vi "Test Status Correct on Added Method.vi"(8 "error in (no error)":errorcluster, 11 "Result Model Tests in":refnum<class "Result Model Test Enumeration.lvclass">) -> (0 "error out":errorcluster, 3 "Result Model Tests out":refnum<class "Result Model Test Enumeration.lvclass">)   [LabVIEW 2020, in "Result Model Test Enumeration.lvclass"]
uses:
  Result Model Test Enumeration.lvclass
  source/User Interface/Result Model/Result Model.lvclass
  206db1ee-aa99-40b9-8881-171f2a77c34b.vi
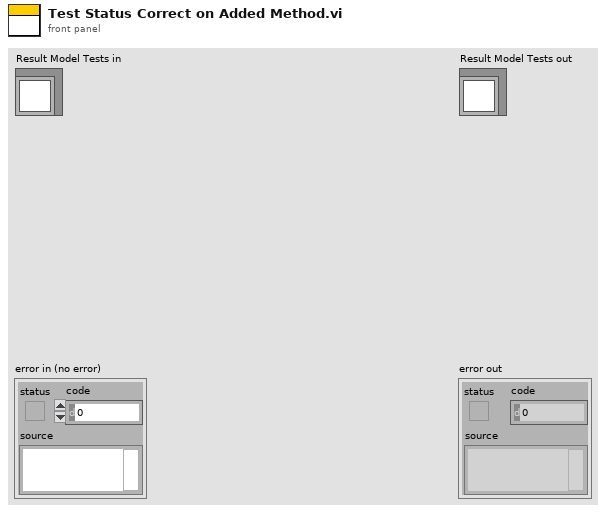
[diagram p1: front panel]
types:
  T1 = cluster{"Left Cell String":string, "Child Text":string[], "Child Tag":string, "Item Indent":i32, "Child Only?":bool, "Glyph Index":i32}[]
  T2 = cluster{"Left Cell String":string, "Child Text":string[], "Child Tag":string, "Item Indent":i32, "Child Only?":bool, "Glyph Index":i32}
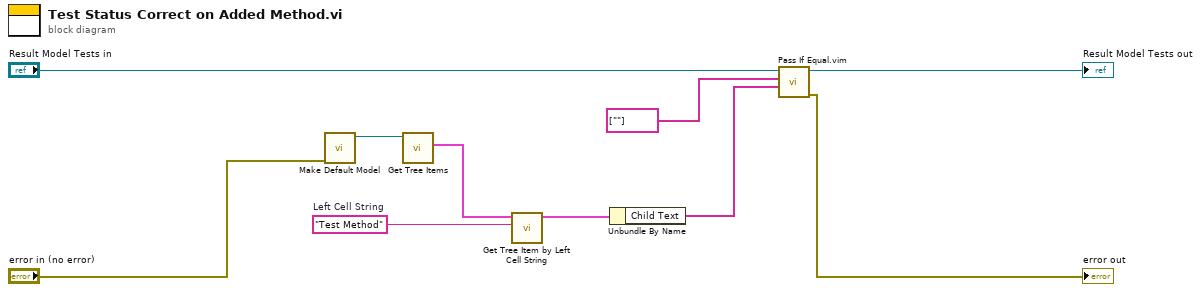
[diagram p0: block diagram]
diagram:
  w2 = "Test Method"  # Left Cell String
  n1 = call "Make Default Model.vi"("error in (no error)"="error in (no error)") -> ("Result Model out"=w9:refnum<class "Result Model.lvclass">)  [unwired: 9 in, 1 out]
  n2 = call "Get Tree Items.vi"("Result Model by Reference In"=w9) -> ("Tree Items"=w7:T1)  [unwired: 9 in, 1 out]
  n3 = call "Get Tree Item by Left Cell String.vi"("Left Cell String"=w2, "Tree Items"=w7) -> ("Item"=w5:T2)  [unwired: 9 in]
  n4 = Unbundle By Name(w5) -> ("Child Text"=w4:string[])
  n5 = call "Pass If Equal.vim"("Actual"=w4, "Expected"=string[] [""] ("Child Text"), "LUnit Test Case In"="Result Model Tests in") -> ("error out"=→"error out":errorcluster, "LUnit Test Case Out"=→"Result Model Tests out":refnum<class "Result Model Test Enumeration.lvclass">)  [unwired: 7 in]
